vi "_ConvertMassRanges.vi"(7 "ExptParamAndMR":T4) -> (3 "MassRanges":T1[](array[typedef]) {"Res" items=["High/High", "Medium/Medium", "Low/Low", "High/Medium", "High/Low", "Medium/High", "Medium/Low", "Low/High", "Low/Medium"]})   [LabVIEW 2015]
uses:
  Type/_Mass Range Parameters.ctl
  Type/_Mass Range Property.ctl
  Type/_RT Res Type.ctl
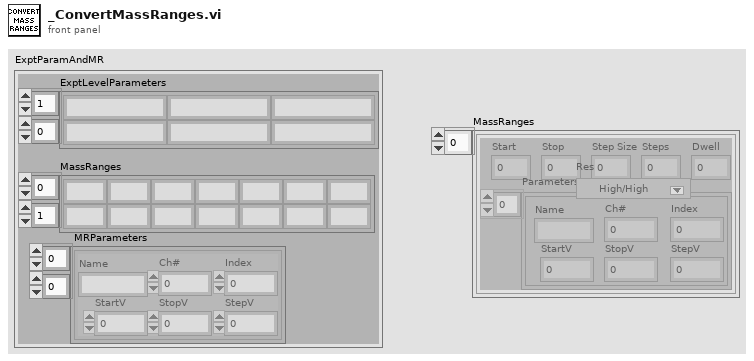
[diagram p1: front panel]
types:
  T1 = typedef "_Mass Range Property.ctl" = cluster{"Start":dbl, "Stop":dbl, "Step Size":dbl, "Steps":i32, "Dwell":dbl, "Parameters":T2[], "Res":T3}
  T2 = typedef "_Mass Range Parameters.ctl" = cluster{"Name":string, "Ch#":u8, "StartV":dbl, "StopV":dbl, "StepV":dbl, "Index":u8}
  T3 = typedef "_RT Res Type.ctl" = u16
  T4 = cluster{"ExptLevelParameters":string[][], "MassRanges":string[][], " MRParameters":T2[][]}
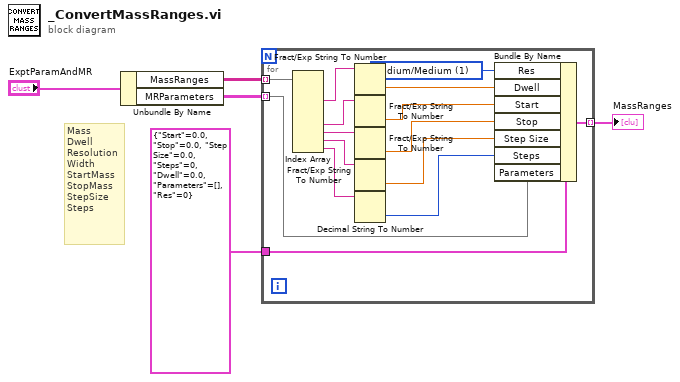
[diagram p0: block diagram]
diagram:
  # "Mass\nDwell\nResolution\nWidth\nStartMass\nStopMass\nStepSize\nSteps"
  n1 = Unbundle By Name("ExptParamAndMR") -> ("MassRanges"=w4:string[][], "MRParameters"=w3:T2[][])
  n2 = for {
    tunnel: w4 -> [w20] mode=indexing
    tunnel: w3 -> [w7] mode=indexing
    tunnel: T1 {"Start"=0.0, "Stop"=0.0, "Step Size"=0.0, "Steps"=0, "Dwell"=0.0, "Parameters"=[], "Res"=0} ("Mass Range") -> [w14]
    tunnel: [w6] -> w1 mode=indexing
    w8 = T3 1 items=["High/High", "Medium/Medium", "Low/Low", "High/Medium", "High/Low", "Medium/High", "Medium/Low", "Low/High", "Low/Medium"] ("Res")
    n3 = Index Array(array=w20) -> (element #2=w17:string, element #5=w19:string, element #6=w18:string, element #7=w16:string, element #8=w15:string)  [unwired: 8 in, 3 out]
    n4 = Fract/Exp String To Number(string=w17) -> (number=w12:dbl)  [unwired: 3 in, 1 out]
    n5 = Fract/Exp String To Number(string=w19) -> (number=w11:dbl)  [unwired: 3 in, 1 out]
    n6 = Fract/Exp String To Number(string=w18) -> (number=w10:dbl)  [unwired: 3 in, 1 out]
    n7 = Fract/Exp String To Number(string=w16) -> (number=w9:dbl)  [unwired: 3 in, 1 out]
    n8 = Decimal String To Number(string=w15) -> (number=w13:i32)  [unwired: 2 in, 1 out]
    n9 = Bundle By Name(cluster=w14, "Res"=w8, "Dwell"=w12, "Start"=w11, "Stop"=w10, "Step Size"=w9, "Steps"=w13, "Parameters"=w7) -> (w6:T1)
  }
  "MassRanges" <- w1
